vi "Post-Build Custom Action.vi"(10 "Variant":variant) -> (0 "error out":errorcluster)   [LabVIEW 2016]
uses:
  PostBuildSupport/PostBuildSupport.lvclass
  PostBuildSupport/PostBuildSupport.lvclass/PostBuildSupport.ctl
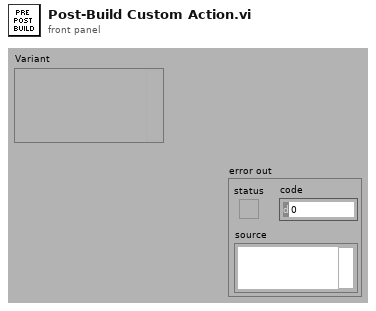
[diagram p1: front panel]
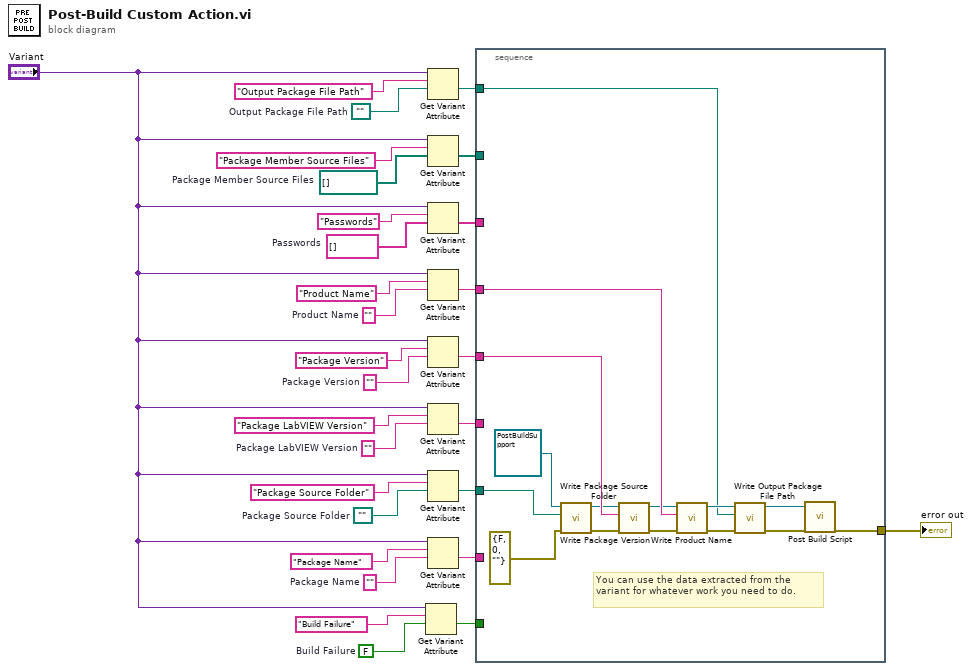
[diagram p0: block diagram]
diagram:
  w4 = FALSE  # Build Failure
  w14 = path ""  # Package Source Folder
  w15 = ""  # Package Name
  w18 = ""  # Package LabVIEW Version
  w20 = ""  # Package Version
  w22 = ""  # Product Name
  w24 = string[] []  # Passwords
  w26 = path[] []  # Package Member Source Files
  w28 = path ""  # Output Package File Path
  n1 = Get Variant Attribute(Variant="Variant", name="Build Failure", default value (empty Variant)=w4) -> (value=w2:bool)  [unwired: 1 in, 3 out]
  n2 = Get Variant Attribute(Variant="Variant", name="Output Package File Path", default value (empty Variant)=w28) -> (value=w13:path)  [unwired: 1 in, 3 out]
  n3 = Get Variant Attribute(Variant="Variant", name="Package Member Source Files", default value (empty Variant)=w26) -> (value=w12:path[])  [unwired: 1 in, 3 out]
  n4 = Get Variant Attribute(Variant="Variant", name="Passwords", default value (empty Variant)=w24) -> (value=w11:string[])  [unwired: 1 in, 3 out]
  n5 = Get Variant Attribute(Variant="Variant", name="Product Name", default value (empty Variant)=w22) -> (value=w10:string)  [unwired: 1 in, 3 out]
  n6 = Get Variant Attribute(Variant="Variant", name="Package Version", default value (empty Variant)=w20) -> (value=w9:string)  [unwired: 1 in, 3 out]
  n7 = Get Variant Attribute(Variant="Variant", name="Package LabVIEW Version", default value (empty Variant)=w18) -> (value=w8:string)  [unwired: 1 in, 3 out]
  n8 = Get Variant Attribute(Variant="Variant", name="Package Source Folder", default value (empty Variant)=w14) -> (value=w7:path)  [unwired: 1 in, 3 out]
  n9 = Get Variant Attribute(Variant="Variant", name="Package Name", default value (empty Variant)=w15) -> (value=w6:string)  [unwired: 1 in, 3 out]
  n10 = stacked-sequence {
    tunnel: w13 -> [w30]
    tunnel: w12 -> [_]
    tunnel: w11 -> [_]
    tunnel: w10 -> [w42]
    tunnel: w9 -> [w43]
    tunnel: w8 -> [_]
    tunnel: w7 -> [w32]
    tunnel: w6 -> [_]
    tunnel: w2 -> [_]
    tunnel: [w44] -> w1
    frame #0 {
      # "You can use the data extracted from the variant for whatever work you need to do."
      n11 = call "Write Package Source Folder.vi"("error in (no error)"=errorcluster {"status"=FALSE, "code"=0, "source"=""} ("error in"), "Package Source Folder"=w32, "PostBuildSupport in"=refnum<class "PostBuildSupport.lvclass"> refnum) -> ("error out"=w39:errorcluster, "PostBuildSupport out"=w40:refnum<class "PostBuildSupport.lvclass">)  [unwired: 7 in]
      n12 = call "Write Package Version.vi"("error in (no error)"=w39, "Package Version"=w43, "PostBuildSupport in"=w40) -> ("error out"=w37:errorcluster, "PostBuildSupport out"=w38:refnum<class "PostBuildSupport.lvclass">)  [unwired: 7 in]
      n13 = call "Write Product Name.vi"("error in (no error)"=w37, "Product Name"=w42, "PostBuildSupport in"=w38) -> ("error out"=w35:errorcluster, "PostBuildSupport out"=w36:refnum<class "PostBuildSupport.lvclass">)  [unwired: 7 in]
      n14 = call "Write Output Package File Path.vi"("error in (no error)"=w35, "Output Package File Path"=w30, "PostBuildSupport in"=w36) -> ("error out"=w33:errorcluster, "PostBuildSupport out"=w34:refnum<class "PostBuildSupport.lvclass">)  [unwired: 7 in]
      n15 = call "Post Build Script.vi"("PostBuildSupport in"=w34, "error in (no error)"=w33) -> ("error out"=w44:errorcluster)  [unwired: 17 in]
    }
  }
  "error out" <- w1
